vi "http set response header.vi"(7 "override?":bool, 9 "header field data":string, 10 "header field name":string, 11 "application request in":T1) -> (3 "application request out":T1)   [LabVIEW 2016, in "Basic HTTPS server.lvclass"]
uses:
  Basic HTTPS server.lvclass
  http response.ctl
  HTTP headers/http header data.ctl
  HTTP headers/http headers.lvlib
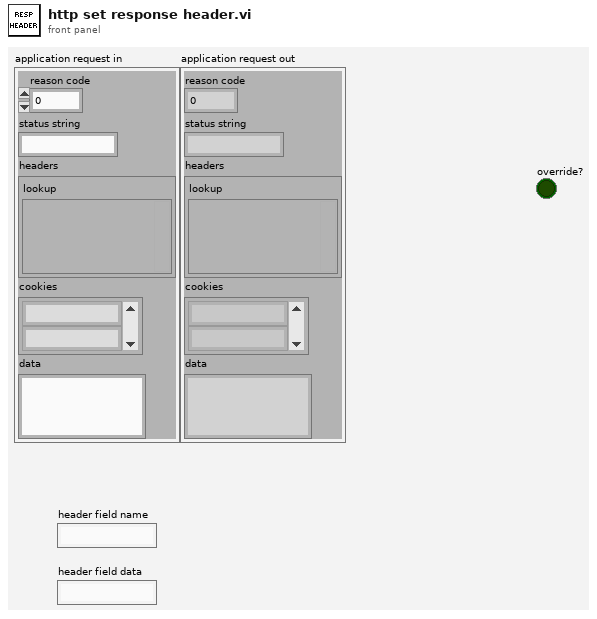
[diagram p1: front panel]
types:
  T1 = typedef "Basic HTTPS server.lvclass/http response.ctl" = cluster{"reason code":u16, "status string":string, "headers":T2, "cookies":string[], "data":string}
  T2 = typedef "http headers.lvlib/http header data.ctl" = cluster{"lookup":variant}
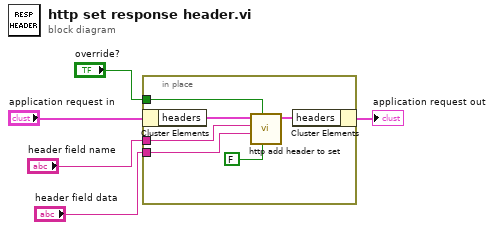
[diagram p0: block diagram]
diagram:
  n1 = in-place {
    in-place-border: "header field name" -> [w9]
    in-place-border: "header field data" -> [w8]
    in-place-border: "override?" -> [w10]
    n2 = in-place-cluster #1("application request in") -> ("headers"=w11:T2)
    n3 = call "http add header to set.vi"("continuation?"=FALSE, "override on duplicate?"=w10, "header field data"=w8, "header field name"=w9, "headers in"=w11) -> ("headers out"=w6:T2)  [unwired: 6 in]
    n4 = in-place-cluster #1("headers"=w6) -> (→"application request out":T1)
  }
